vi "UI_Resize.vi"(8 "error in (no error)":errorcluster, 11 "D&C_SchemaBase in":refnum<class "D&C_SchemaBase.lvclass">) -> (0 "error out":errorcluster, 3 "D&C_SchemaBase out":refnum<class "D&C_SchemaBase.lvclass">)   [LabVIEW 2020, in "D&C_SchemaBase.lvlib" / "D&C_SchemaBase.lvclass"]
uses:
  D&C_SchemaBase.lvclass
  D:/Projets/STEP AT/LUGE 2022.2/UIA_Demo/support/UI_Actor.lvlibp/UI_Actor/UI_Actor.lvclass
  support/Window Toolkit.lvlibp/1abvi3w/vi.lib/Utility/miscctls.llb/LVPointTypeDef.ctl
  support/UI_Actor.lvlibp/UI_Actor/Read CoreRef.vi
  support/UI_Actor.lvlibp/UI_Actor/UI_Actor.lvclass
  support/Window Toolkit.lvlibp
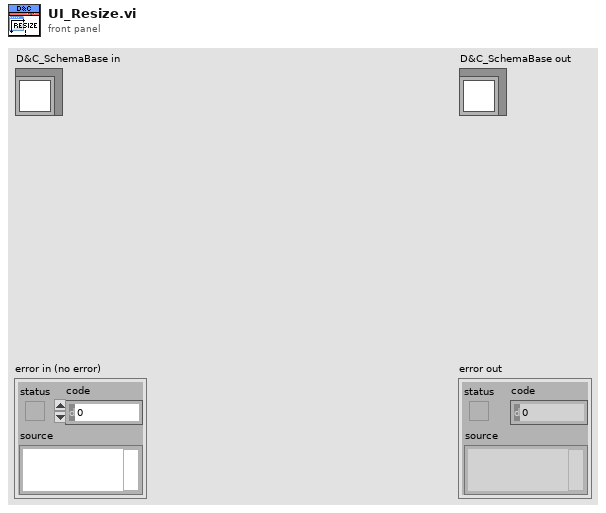
[diagram p1: front panel]
types:
  T1 = typedef "Window Toolkit.lvlibp/LVPointTypeDef.ctl" = cluster{"Horizontal":i16, "Vertical":i16}
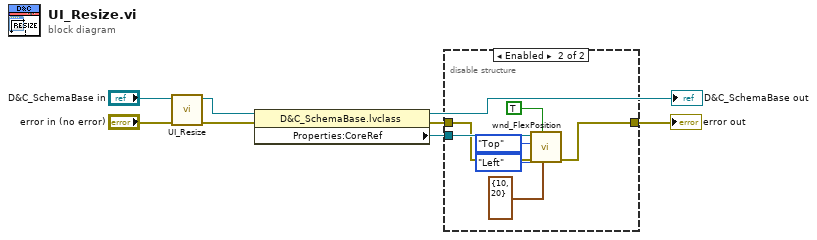
[diagram p0: block diagram]
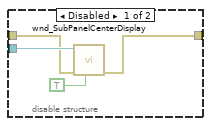
[diagram p2: hidden frame]
diagram:
  n1 = call-parent "UI_Resize.vi"("error in (no error)"="error in (no error)", "UI_Actor in"="D&C_SchemaBase in") -> ("error out"=w6:errorcluster, "UI_Actor out"=w5:refnum<class "D&C_SchemaBase.lvclass">)  [unwired: 8 in]
  n2 = property class="D&C_SchemaBase.lvclass"(reference=w5, error in=w6) -> (reference out=→"D&C_SchemaBase out":refnum<class "D&C_SchemaBase.lvclass">, error out=w2:errorcluster, "Properties:CoreRef"=w3:refnum<vi>)
  n3 = disable-structure shown="Enabled" {
    disable-tunnel: w3 -> [w12 w18]
    disable-tunnel: w2 -> [w10 w17]
    disable-tunnel: [w9 w16] -> w1
    frame Disabled {
      n4 = call "wnd_SubPanelCenterDisplay.vi"("Show scroll if too small"=TRUE, "error in (no error)"=w10, "VI ref"=w12) -> ("error out"=w9:errorcluster)  [unwired: 7 in, 1 out]
    }
    frame Enabled {
      n5 = call "wnd_FlexPosition.vi"("Margin"=T1 {"Horizontal"=10, "Vertical"=20} ("Origin"), "Show scroll if too small"=TRUE, "error in (no error)"=w17, "Justification"=enum16{"Left", "Center", "Right"}."Left", "Alignment"=enum16{"Top", "Center", "Bottom"}."Top", "VI ref"=w18) -> ("error out"=w16:errorcluster)  [unwired: 4 in, 1 out]
    }
  }
  "error out" <- w1
